vi "SystemLink_RESTful.vi"(6 "Method":T2(ring), 7 "url":string, 8 "error in":errorcluster, 9 "data":T1[](array[typedef]), 10 "JSON":string, 11 "Device In":T4={"Name"="", "BaseURL"="", "AppKey"="", "Headers"=["Content-Type:application/json"], "Timeout"=10000}) -> (0 "error out":errorcluster, 1 "HTTP Code":i32, 2 "Comm":T3, 3 "Device Out":T4={"Name"="", "BaseURL"="", "AppKey"="", "Headers"=["Content-Type:application/json"], "Timeout"=10000})   [LabVIEW 2016]
uses:
  <vilib>/httpClient/LabVIEWHTTPClient.lvlib
  <vilib>/httpClient/PUTBuffer.vi
  <vilib>/httpClient/POSTBuffer.vi
  SkylineCluster.ctl
  SystemLinkHTTPComm.ctl
  <vilib>/httpClient/MultipartData.ctl
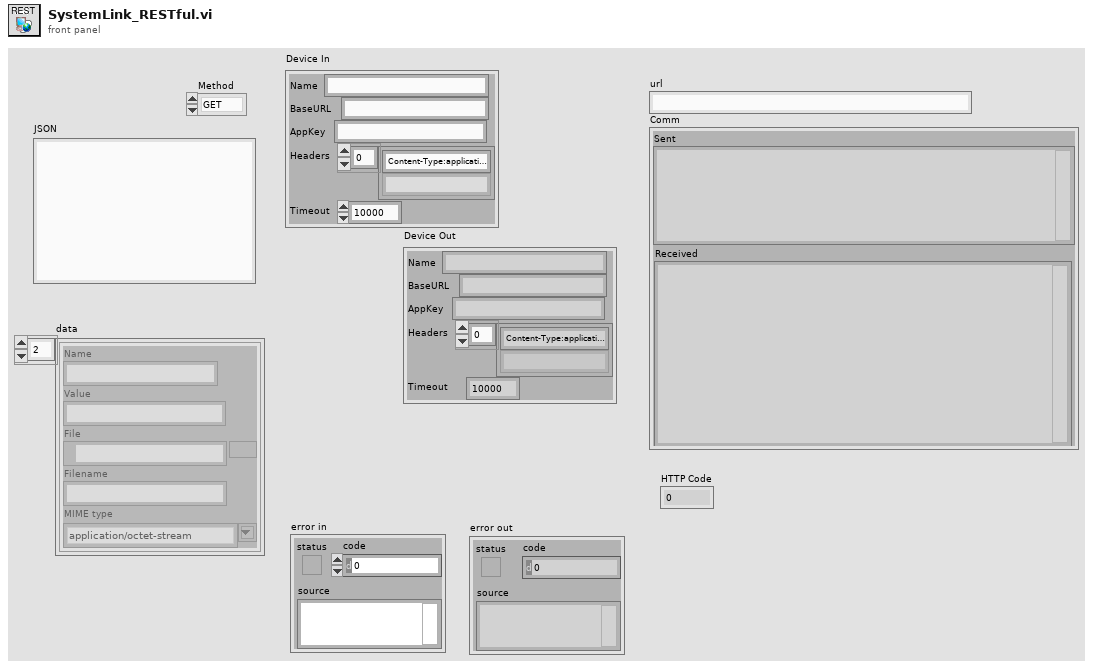
[diagram p1: front panel]
types:
  T1 = typedef "LabVIEWHTTPClient.lvlib/MultipartData.ctl" = cluster{"Name":string, "Value":string, "File":path, "Filename":string, "MIME type":string}
  T2 = enum16{"GET", "PUT", "POST", "MultiPOST", "DELETE"}
  T3 = typedef "SystemLinkHTTPComm.ctl" = cluster{"url":string, "sent headers":string, "sent body":string, "headers":string, "body":string, "Sent":string, "Received":string}
  T4 = typedef "SkylineCluster.ctl" = cluster{"Name":string, "BaseURL":string, "AppKey":string, "Headers":string[], "Timeout":i32}
  T5 = typedef "LabVIEWHTTPClient.lvlib/ClientHandle.ctl" = refnum<k1>
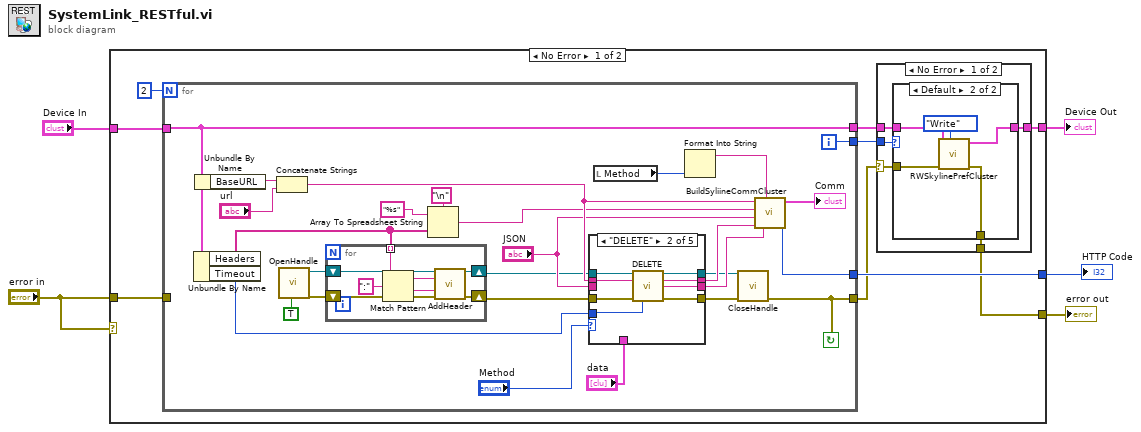
[diagram p0: block diagram]
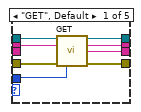
[diagram p4: hidden frame]
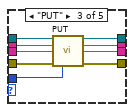
[diagram p5: hidden frame]
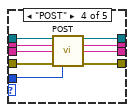
[diagram p6: hidden frame]
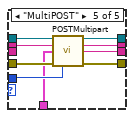
[diagram p7: hidden frame]
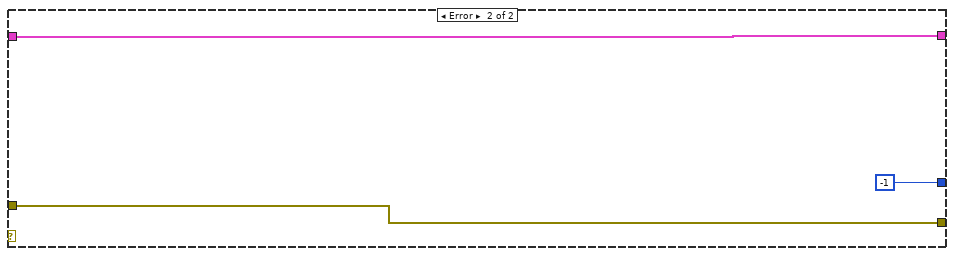
[diagram p8: hidden frame]
diagram:
  n1 = case shown="No Error" "error in" {
    tunnel: "error in" -> [w12 w108]
    tunnel: "Device In" -> [w11 w109]
    tunnel: [w8 w109] -> w4
    tunnel: [w6 w108] -> w3
    tunnel: [w14 -1 ("error")] -> w1
    frame No Error {
      n2 = for {
        N: 2 -> [_]
        tunnel: [w33] -> w14
        tunnel: w12 -> [_]
        tunnel: [w29] -> w7
        tunnel: [w41] -> w9
        tunnel: w11 -> [w41]
        tunnel: [w45] -> w10
        i -> [w45]
        stop <- w29 continue-if-true
        n3 = Unbundle By Name(w41) -> ("Headers"=w39:string[], "Timeout"=w40:i32)
        n4 = Unbundle By Name(w41) -> ("BaseURL"=w51:string)
        n5 = Concatenate Strings(w51, "url") -> (w54:string)
        n6 = call <vilib>:"OpenHandle.vi"("verify server(true)"=TRUE) -> ("client handle out"=w43:T5, "error out"=w44:errorcluster)  [unwired: 13 in]
        n7 = for {
          shift-right: [w62] -> w35
          shift-left: w43 -> [w63]
          shift-right: [w60] -> w34
          shift-left: w44 -> [w61]
          tunnel: w39 -> [w56] mode=indexing
          n8 = Match Pattern(string=w56, regular expression=":") -> (before substring=w58:string, after substring=w57:string)  [unwired: 1 in, 2 out]
          n9 = call <vilib>:"AddHeader.vi"("client handle"=w63, "header"=w58, "value"=w57, "error in (no error)"=w61) -> ("client handle out"=w62:T5, "error out"=w60:errorcluster)  [unwired: 10 in]
        }
        n10 = Array To Spreadsheet String(delimiter (Tab)="\n", array=w39, 3:"%s" ("format string")) -> (spreadsheet string=w36:string)
        n11 = case shown="\"DELETE\"" "Method" {
          tunnel: [w71 w79 w88 w97 w106] -> w55
          tunnel: [w70 w78 w87 w96 w105] -> w32
          tunnel: [w69 w77 w86 w95 w104] -> w30
          tunnel: w40 -> [w68 w76 w85 w94 w103]
          tunnel: w54 -> [w67 w75 w84 w93 w102]
          tunnel: w34 -> [w66 w74 w83 w92 w101]
          tunnel: w35 -> [w65 w73 w82 w91 w100]
          tunnel: "JSON" -> [_ _ w81 w90 _]
          tunnel: [w64 w72 w80 w89 w99] -> w31
          tunnel: "data" -> [_ _ _ _ w98]
          frame "GET", Default {
            n12 = call <vilib>:"GET.vi"("client handle"=w65, "url"=w67, "error in (no error)"=w66, "timeout (10000)"=w68) -> ("client handle out"=w64:T5, "headers"=w71:string, "body"=w70:string, "error out"=w69:errorcluster)  [unwired: 8 in]
          }
          frame "DELETE" {
            n13 = call <vilib>:"DELETE.vi"("client handle"=w73, "url"=w75, "error in (no error)"=w74, "timeout (10000)"=w76) -> ("client handle out"=w72:T5, "headers"=w79:string, "body"=w78:string, "error out"=w77:errorcluster)  [unwired: 8 in]
          }
          frame "PUT" {
            n14 = call-poly <vilib>:"PUT.vi"("client handle"=w82, "url"=w84, "buffer"=w81, "error in (no error)"=w83, "timeout (10000)"=w85) -> ("client handle out"=w80:T5, "headers"=w88:string, "body"=w87:string, "error out"=w86:errorcluster)  [unwired: 7 in]
          }
          frame "POST" {
            n15 = call-poly <vilib>:"POST.vi"("client handle"=w91, "url"=w93, "buffer"=w90, "error in (no error)"=w92, "timeout (10000)"=w94) -> ("client handle out"=w89:T5, "headers"=w97:string, "body"=w96:string, "error out"=w95:errorcluster)  [unwired: 7 in]
          }
          frame "MultiPOST" {
            n16 = call <vilib>:"POSTMultipart.vi"("client handle"=w100, "url"=w102, "data"=w98, "error in (no error)"=w101, "timeout (10000)"=w103) -> ("client handle out"=w99:T5, "headers"=w106:string, "body"=w105:string, "error out"=w104:errorcluster)  [unwired: 7 in]
          }
        }
        n17 = local read "Method"() -> (w49:T2)
        n18 = Format Into String(w49) -> (resulting string=w48:string)  [unwired: 3 in, 1 out]
        n19 = call <vilib>:"CloseHandle.vi"("client handle"=w31, "error in (no error)"=w30) -> ("error out"=w29:errorcluster)  [unwired: 13 in]
        n20 = call "BuildSyliineCommCluster.vi"("reply body"=w32, "Type"=w48, "reply headers"=w55, "sent body"="JSON", "sent headers"=w36, "url"=w54) -> ("Code"=w33:i32, "Comm"=→"Comm":T3)  [unwired: 4 in]
      }
      n21 = case shown="No Error" w7 {
        selector: w7 -> [w15 w27]
        tunnel: w10 -> [w19 _]
        tunnel: w9 -> [w18 w28]
        tunnel: [w17 w28] -> w8
        tunnel: [w16 w27] -> w6
        frame No Error {
          n22 = case shown="Default" w19 {
            tunnel: w18 -> [w21 w26]
            tunnel: [w21 w24] -> w17
            tunnel: [w20 w22] -> w16
            tunnel: w15 -> [w20 w23]
            frame 0 {
            }
            frame Default {
              n23 = call "RWSkylinePrefCluster.vi"("Task"=enum16{"Read", "Write"}."Write", "error in (no error)"=w23, "Device In"=w26) -> ("error out"=w22:errorcluster, "Device Out"=w24:T4)  [unwired: 7 in]
            }
          }
        }
        frame Error {
        }
      }
    }
    frame Error {
    }
  }
  "error out" <- w3
  "Device Out" <- w4
  "HTTP Code" <- w1
